vi "Current Position Read.vi"(4 "error in (no error)":errorcluster, 6 "Container State":T2, 7 "Display State In":T1) -> (0 "error out":errorcluster, 2 "Value":i32, 3 "Display State Out":T1)   [LabVIEW 2012, in "Waveform Control.xctl"]
doc: "Returns the index of the current position marker. If the current position marker is not visible, then returns -1"
uses:
  Waveform Control.xctl
  <vilib>/_xctls/Container State.ctl
  Controls/State.ctl
  Controls/Volatile State Ops.ctl
  <vilib>/_xctls/XControlSupport.lvlib
panel:
  # "Replace the Value Indicator below with an Indicator of desired type.\nDo not remove this Indicator or the others from the connector pane. \nDo not change the connector pane pattern.\nThe Value Indicator should always be the second terminal from top on the output side in the connector pane."
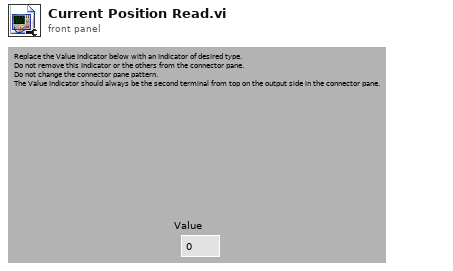
[diagram p1: front panel]
types:
  T1 = typedef "Waveform Control.xctl/State.ctl" = cluster{"Name":string}
  T2 = typedef "XControlSupport.lvlib/Container State.ctl" = cluster{"Indicator?":bool, "Run Mode?":bool, " Refnum":refnum<vi>}
  T3 = typedef "Waveform Control.xctl/Volatile State Ops.ctl" = enum16{"Read", "Write", "Update State from Data"}
  T4 = typedef "Waveform Control.xctl/Waveform State.ctl" = cluster{"Show Axes":bool, "Show Y=0":bool, "Controls":T5, "Show Current Location":bool, "Current Location":i32, "dt":dbl, "t0":timestamp, "Amplitude Format String":string}
  T5 = typedef "Waveform Control.xctl/FP Controls.ctl" = cluster{"Type":T6, "Periods":dbl, "Points":i32, "Offset":dbl, "Amplitdue":dbl, "Starting Phase":dbl, "func":string}
  T6 = typedef "Waveform Control.xctl/Function Types.ctl" = enum16{"Level", "Sine", "Triangle", "Ramp", "Saw Tooth", "Square", "Function"}
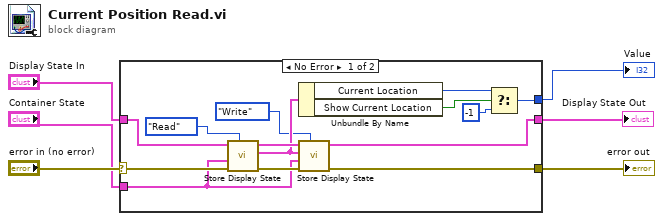
[diagram p0: block diagram]
diagram:
  n1 = case shown="No Error" "error in (no error)" {
    selector: "error in (no error)" -> [w20 w22]
    tunnel: "Display State In" -> [w19 w21]
    tunnel: [w16 w22] -> w3
    tunnel: [w15 w21] -> w5
    tunnel: [w11 _] -> w2
    tunnel: "Container State" -> [w9 _]
    frame No Error {
      n2 = call "Store Display State.vi"("Operation In"=Volatile_State_Ops."Read", "Error In (no Error) In"=w20, "Container State In"=w9, "State In"=w19) -> ("Error Out"=w18:errorcluster, "Waveform State Out"=w14:T4, "Display State Out"=w17:T1)  [unwired: 2 in, 3 out]
      n3 = Unbundle By Name(w14) -> ("Current Location"=w12:i32, "Show Current Location"=w13:bool)
      n4 = call "Store Display State.vi"("Operation In"=Volatile_State_Ops."Write", "Error In (no Error) In"=w18, "Container State In"=w9, "Waveform State In"=w14, "State In"=w17) -> ("Error Out"=w16:errorcluster, "Display State Out"=w15:T1)  [unwired: 1 in, 4 out]
      n5 = Select(t=w12, s=w13, f=-1) -> (s? t:f=w11:i32)
    }
    frame Error {
    }
  }
  "error out" <- w3
  "Value" <- w2
  "Display State Out" <- w5
